vi "test Connect.vi"(8 "error in (no error)":errorcluster, 11 "TestCase in":refnum<class "Test Network Stream Initiator Connect.lvclass">) -> (0 "error out":errorcluster, 3 "TestCase out":refnum<class "Test Network Stream Initiator Connect.lvclass">)   [LabVIEW 2020, in "Test Network Stream Initiator Connect.lvclass"]
uses:
  Test Network Stream Initiator Connect.lvclass
  <vilib>/addons/_JKI Toolkits/VI Tester/TestCase.llb/TestCase.lvclass
  Source/Protocols/Network Stream Strategy/Network Stream Initiator/Network Stream Initiator.lvclass
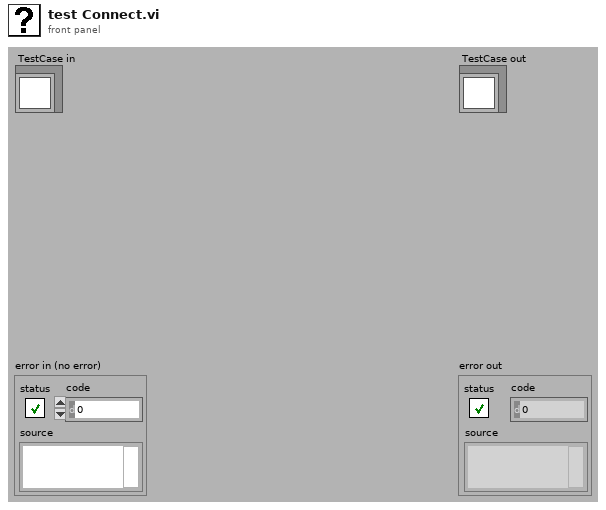
[diagram p1: front panel]
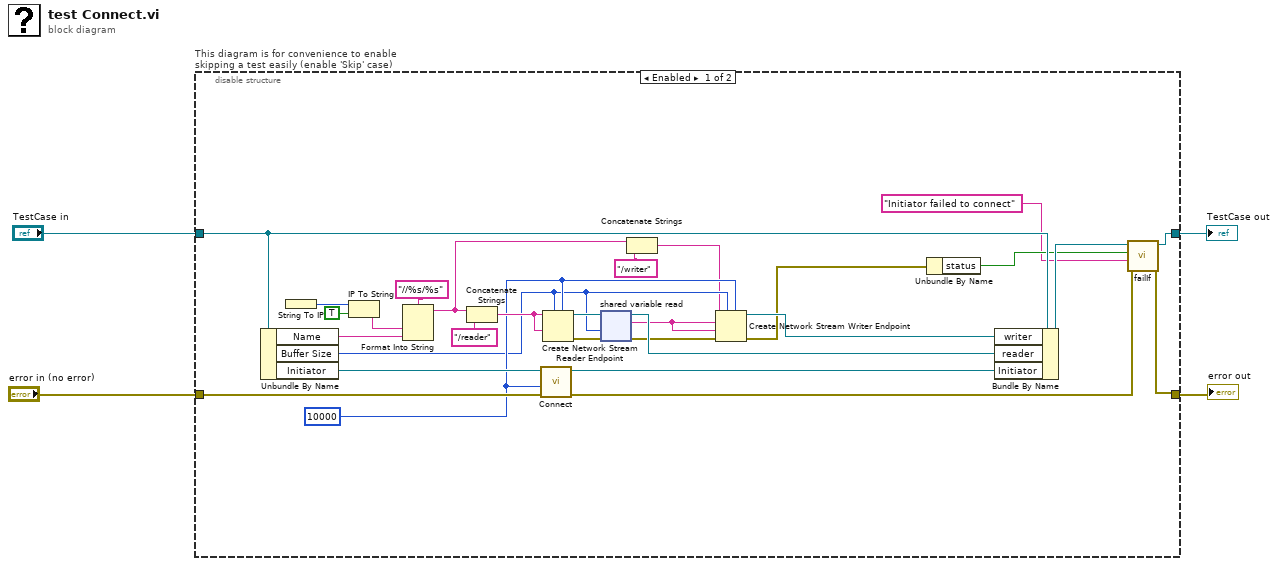
[diagram p0: block diagram]
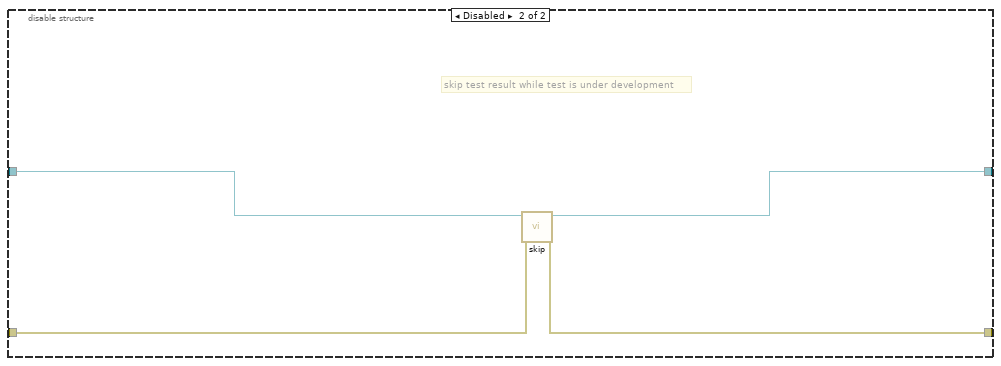
[diagram p2: hidden frame]
diagram:
  n1 = disable-structure "This diagram is for convenience to enable skipping a test easily (enable 'Skip' case)" shown="Enabled" {
    disable-tunnel: "TestCase in" -> [w28 w37]
    disable-tunnel: [w33 w35] -> w1
    disable-tunnel: [w32 w36] -> w3
    disable-tunnel: "error in (no error)" -> [w31 w34]
    frame Enabled {
      w16 = 10000 ("timeout")
      n2 = Unbundle By Name(w28) -> ("Name"=w22:string, "Buffer Size"=w11:i32, "Initiator"=w29:refnum<class "Network Stream Initiator.lvclass">)
      n3 = String To IP() -> (0:w21:u32)  [unwired: 1 in]
      n4 = IP To String(1:TRUE ("dot notation? (F)"), 2:w21) -> (0:w19:string)
      n5 = Format Into String(format string="//%s/%s", w19, w22) -> (resulting string=w6:string)  [unwired: 2 in, 1 out]
      n6 = Concatenate Strings(w6, "/reader" ("format string")) -> (w18:string)
      n7 = call-dynamic "Connect.vi"("error in (no error)"=w31, "timeout"=w16, "Network Stream Initiator in"=w29) -> ("error out"=w30:errorcluster, "Network Stream Initiator out"=w26:refnum<class "Network Stream Initiator.lvclass">)  [unwired: 7 in]
      n8 = Create Network Stream Reader Endpoint(5:w16, 7:w11, 9:w18, 11:w18) -> (0:w13:errorcluster, 3:w12:refnum<k21>)  [unwired: 3 in]
      n9 = shared-variable-read(w12, w13, w11) -> (w10:refnum<k21>, w9:errorcluster, w8:string)  [unwired: 1 out]
      n10 = Concatenate Strings(w6, "/writer" ("format string")) -> (w5:string)
      n11 = Create Network Stream Writer Endpoint(5:w16, 7:w11, 8:w9, 9:w8, 10:w8, 11:w5) -> (0:w14:errorcluster, 3:w15:refnum<k21>)  [unwired: 1 in]
      n12 = Unbundle By Name(w14) -> ("status"=w25:bool)
      n13 = Bundle By Name(cluster=w28, "writer"=w15, "reader"=w10, "Initiator"=w26) -> (w27:refnum<class "Test Network Stream Initiator Connect.lvclass">)
      n14 = call-dynamic "failIf.vi"("error in (no error)"=w30, "message (\"\")"="Initiator failed to connect" ("message (\"\")"), "fail"=w25, "TestCase in"=w27) -> ("error out"=w32:errorcluster, "TestCase out"=w33:refnum<class "Test Network Stream Initiator Connect.lvclass">)  [unwired: 6 in]
    }
    frame Disabled {
      # "skip test result while test is under development"
      n15 = call <vilib>:"skip.vi"("error in (no error)"=w34, "TestCase in"=w37) -> ("error out"=w36:errorcluster, "TestCase out"=w35:refnum<class "Test Network Stream Initiator Connect.lvclass">)  [unwired: 8 in]
    }
  }
  "error out" <- w3
  "TestCase out" <- w1
